vi "LabVIEW Task Manager.vi"() -> ()   [LabVIEW 2013]
doc: "Use this template to create an application that executes until you click the Stop button. Unlike the Single Loop Application VI that uses polling, this VI uses the Event Structure."
panel:
  in  "Data Tree":string[](tree)=["Get File Extension.vi"]
  in  "Timeout (ms)":i32=2000
  in  "vit":bool=TRUE
  in  "vi":bool
  in  "ctl":bool=TRUE
  in  "Open Front Panel":bool
  in  "Open Block Diagram":bool
  in  "Refresh":bool
  in  "Abort":bool
  # "Filter"
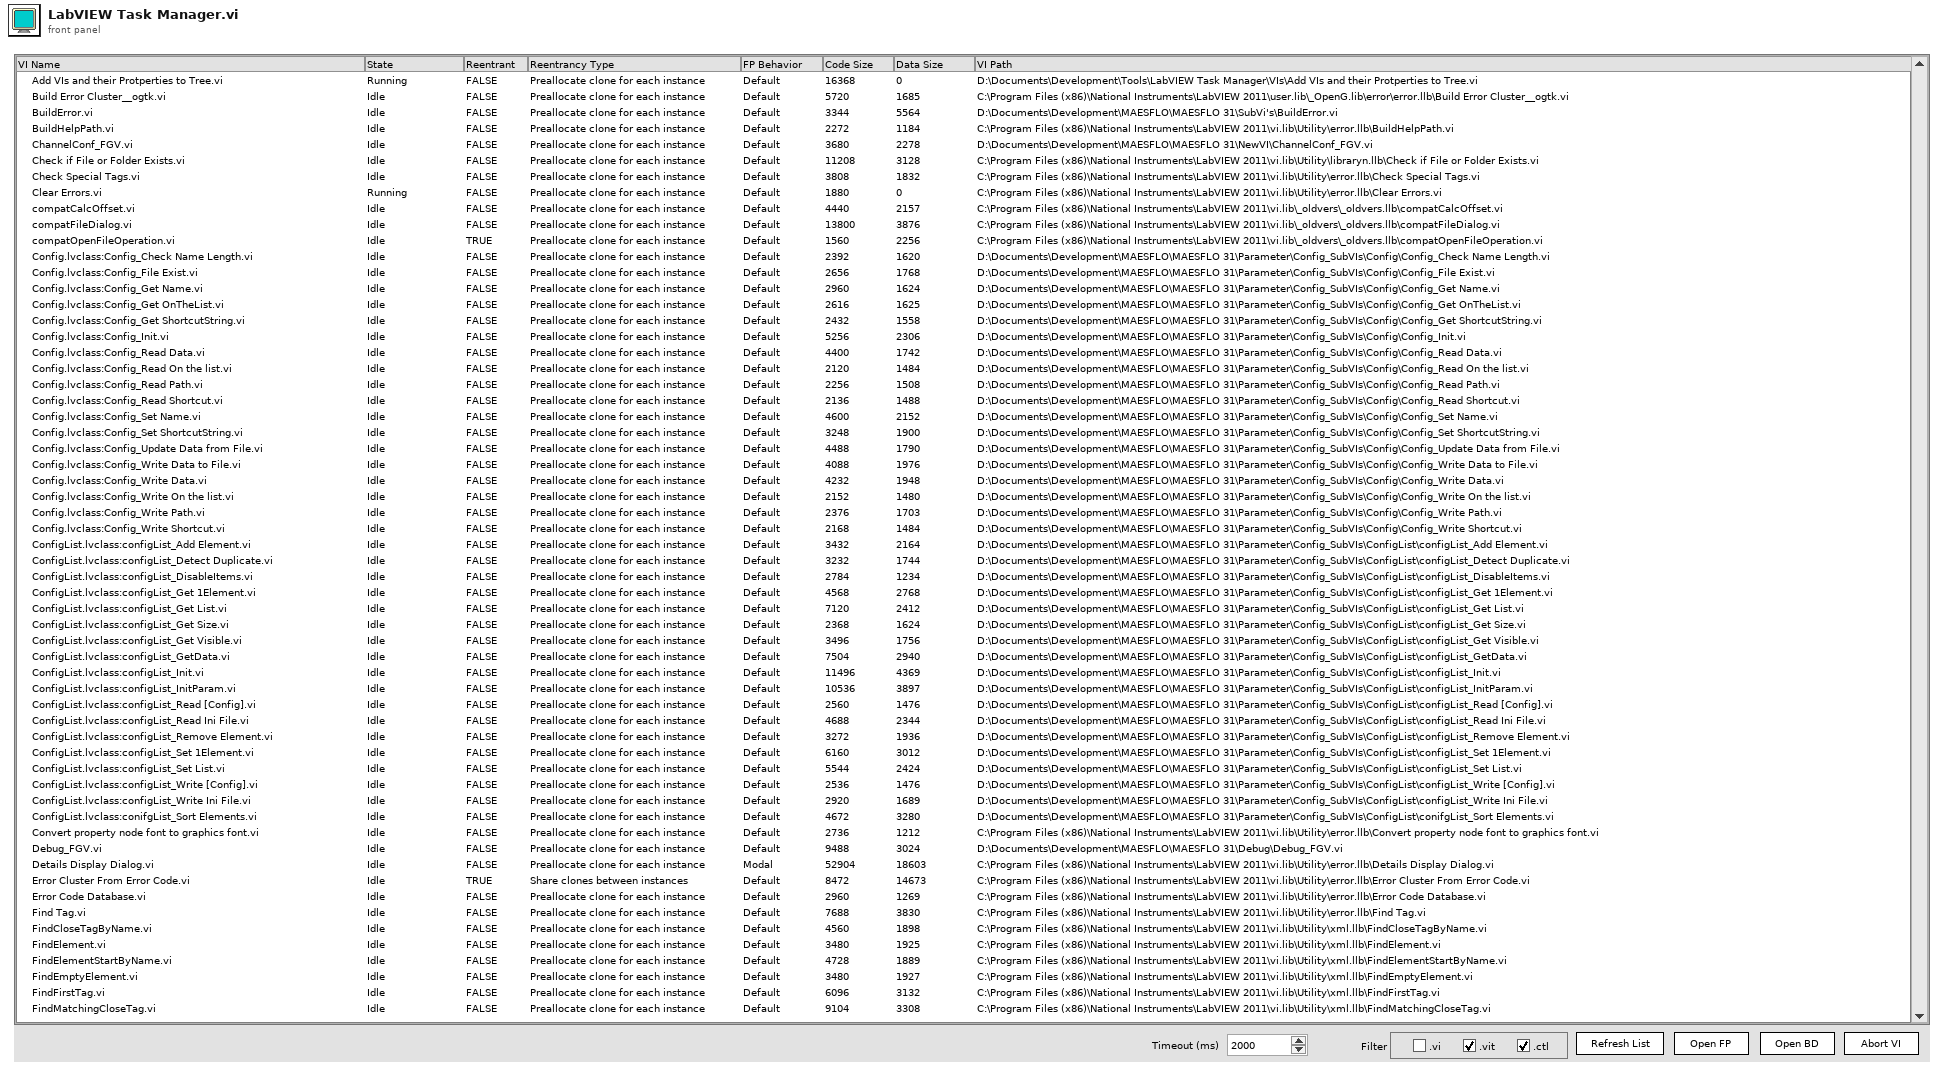
[diagram p1: front panel]
types:
  T1 = cluster{"Sort Column":i32, "Sorted AZ?":bool, "Data Tree Ref":refnum<vi>, "FP Ref":refnum<vi>, "Column Data Type":enum16{"String", "Numeric"}[]}
  T2 = enum32{"Bad", "Idle", "Run top level", "Running"}
  T3 = typedef "LVPoint32TypeDef.ctl" = cluster{"Horizontal":i32, "Vertical":i32}
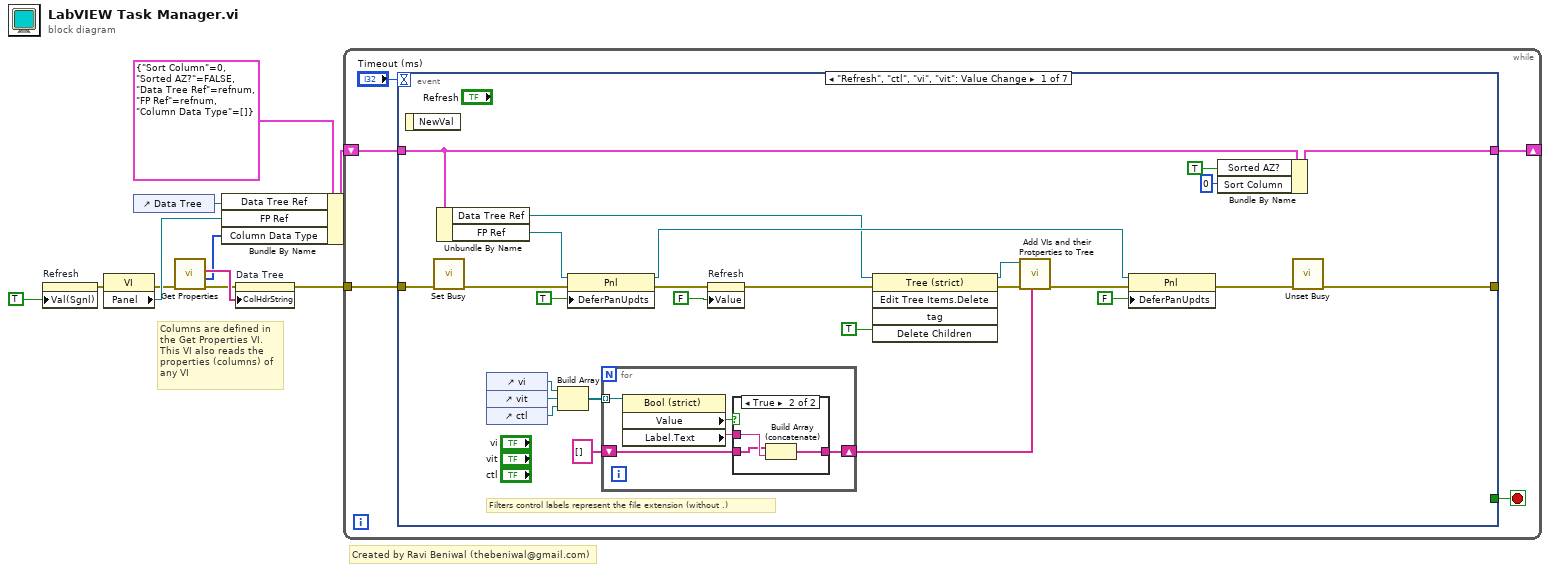
[diagram p0: block diagram]
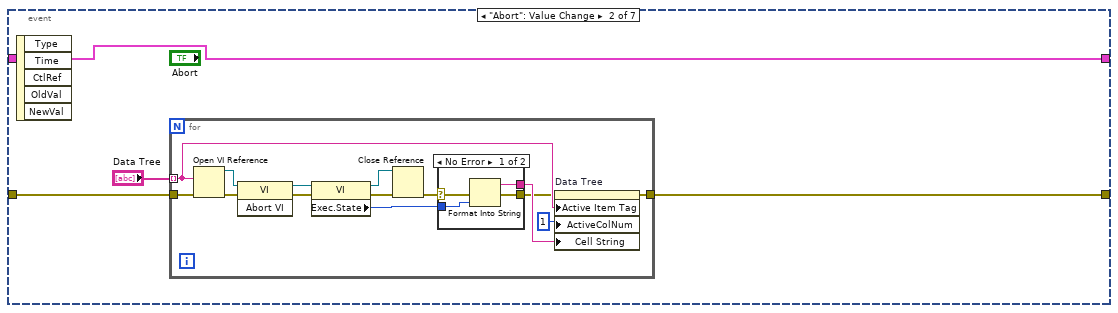
[diagram p3: hidden frame]
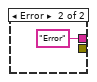
[diagram p4: hidden frame]
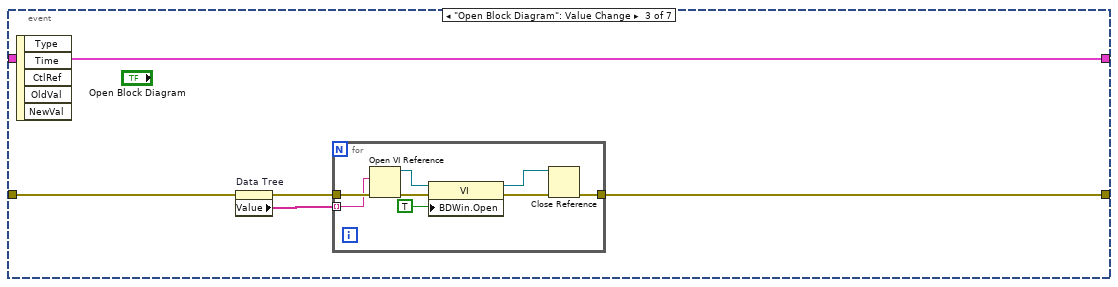
[diagram p5: hidden frame]
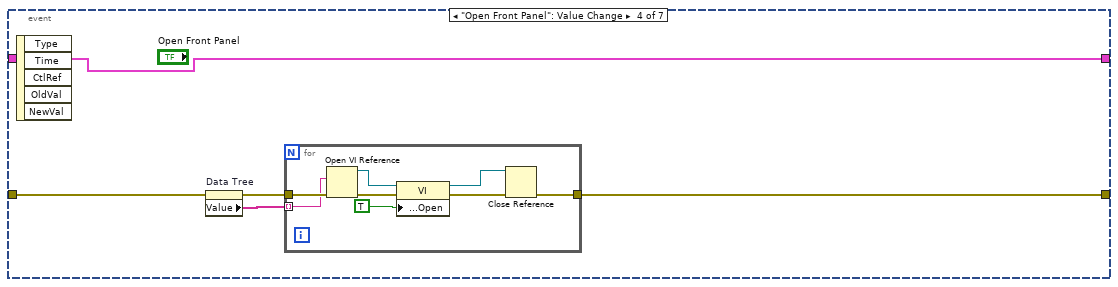
[diagram p6: hidden frame]
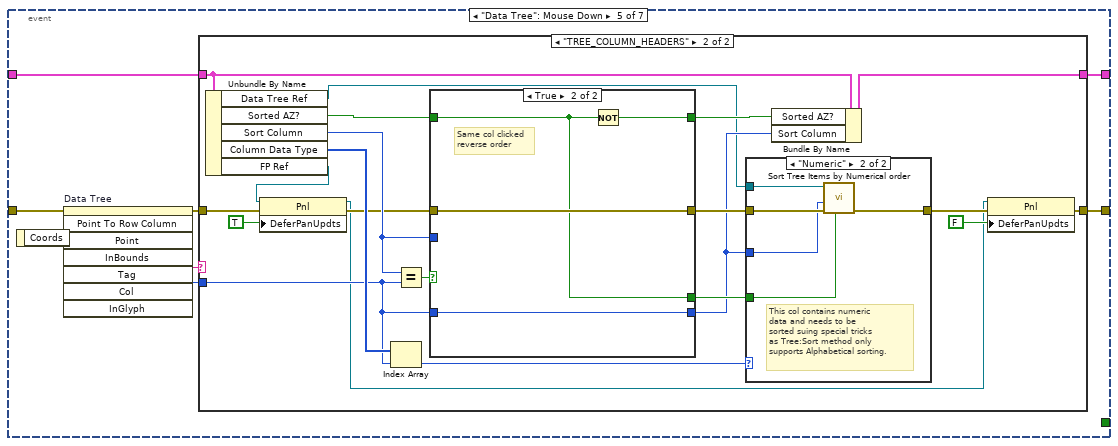
[diagram p7: hidden frame]
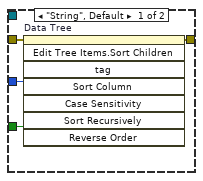
[diagram p9: hidden frame]
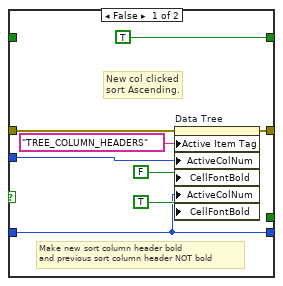
[diagram p10: hidden frame]
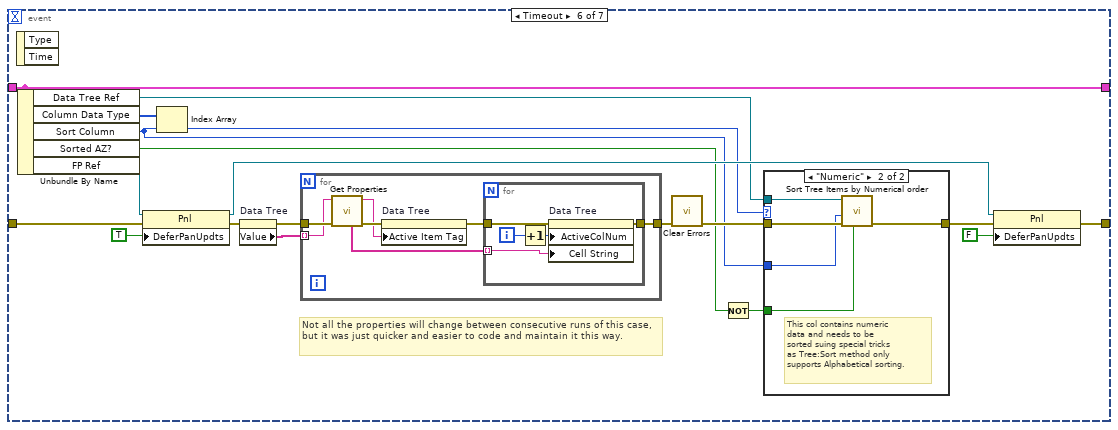
[diagram p11: hidden frame]
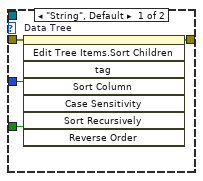
[diagram p12: hidden frame]
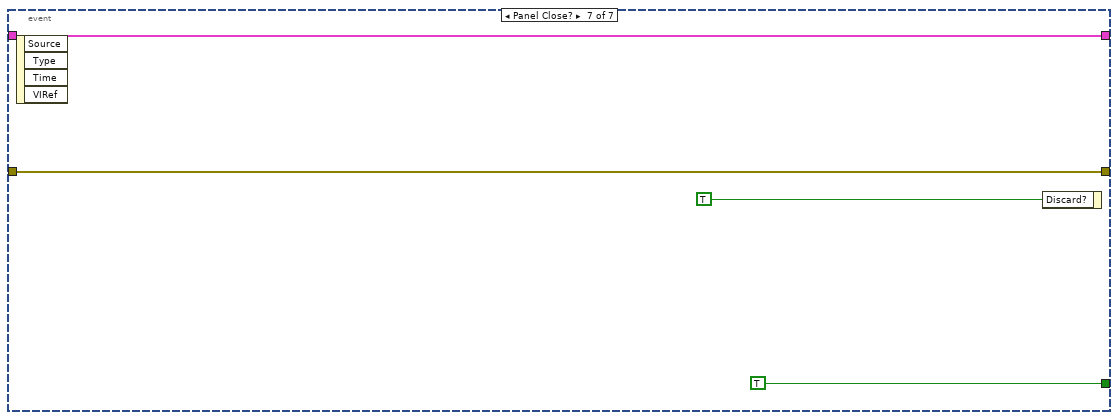
[diagram p13: hidden frame]
diagram:
  # "Columns are defined in the Get Properties VI. This VI also reads the properties (columns) of any VI"
  # "Created by Ravi Beniwal (thebeniwal@gmail.com)"
  n1 = property on="Refresh" class="Bool (strict)"("Val(Sgnl)"=TRUE ("Value (Signaling)")) -> (error out=w4:errorcluster)  [unwired: 2 in, 1 out]
  n2 = property class="VI"(error in=w4) -> (error out=w2:errorcluster, "Panel"=w5:refnum<vi>)  [unwired: 1 in, 1 out]
  n3 = control-ref of="Data Tree"() -> (w8:refnum<vi>)
  n4 = call "Get Properties.vi"("error in"=w2) -> ("error out"=w6:errorcluster, "Column Data Type"=w1:enum16{"String", "Numeric"}[], "Column Labels"=w7:string[])  [unwired: 6 in, 2 out]
  n5 = Bundle By Name(cluster=T1 {"Sort Column"=0, "Sorted AZ?"=FALSE, "Data Tree Ref"=refnum, "FP Ref"=refnum, "Column Data Type"=[]}, "Data Tree Ref"=w8, "FP Ref"=w5, "Column Data Type"=w1) -> (w9:T1)
  n6 = property on="Data Tree" class="Tree (strict)"(error in=w6, "ColHdrString"=w7) -> (error out=w3:errorcluster)  [unwired: 1 in, 1 out]
  n7 = while {
    tunnel: w3 -> [w15]
    shift-right: [w12] -> _
    shift-left: w9 -> [w13]
    stop <- w16 stop-if-true
    n8 = event shown="[0] \"Refresh\", \"ctl\", \"vi\", \"vit\": Value Change" {
      selector: _ -> [_ _ _ _ _ _ _]
      dyn-events: _ -> [_ _ _ _ _ _ _]
      timeout: "Timeout (ms)" -> [_ _ _ _ _ _ _]
      tunnel: [_ _ _ _ _ _ TRUE ("stop")] -> w16
      tunnel: [w33 w55 w78 w91 w103 w165 w195] -> _
      tunnel: w15 -> [w32 w54 w79 w92 w108 w167 w195]
      tunnel: w13 -> [w20 w52 w75 w88 w101 w153 w193]
      tunnel: [w23 w52 w75 w88 w102 w153 w193] -> w12
      event "Refresh", "ctl", "vi", "vit": Value Change {
        # "Filters control labels represent the file extension (without .)"
        n9 = event-data() -> ()  [unwired: 2 out]
        n10 = call <vilib>:"Set Busy.vi"("error in (no error)"=w32) -> ("error out"=w17:errorcluster)  [unwired: 9 in, 1 out]
        n11 = Unbundle By Name(w20) -> ("Data Tree Ref"=w19:refnum<vi>, "FP Ref"=w18:refnum<vi>)
        n12 = control-ref of="vi"() -> (w31:refnum<vi>)
        n13 = control-ref of="vit"() -> (w30:refnum<vi>)
        n14 = control-ref of="ctl"() -> (w29:refnum<vi>)
        n15 = Build Array(w31, w30, w29) -> (w28:refnum<vi>[])
        n16 = property class="Pnl"(reference=w18, error in=w17, "DeferPanUpdts"=TRUE ("Defer Panel Updates")) -> (reference out=w21:refnum<vi>, error out=w35:errorcluster)
        n17 = for {
          tunnel: w28 -> [w47] mode=indexing
          shift-right: [w43] -> w26
          shift-left: string[] [] -> [w44]
          n18 = property class="Bool (strict)"(reference=w47) -> ("Value"=w46:bool, "Label.Text"=w45:string)  [unwired: 1 in, 2 out]
          n19 = case shown="True" w46 {
            tunnel: w45 -> [_ w51]
            tunnel: w44 -> [w48 w50]
            tunnel: [w48 w49] -> w43
            frame False {
            }
            frame True {
              n20 = Build Array (concatenate)(w50, w51) -> (w49:string[])
            }
          }
        }
        n21 = property on="Refresh" class="Bool (strict)"(error in=w35, "Value"=FALSE ("Refresh")) -> (error out=w39:errorcluster)  [unwired: 1 in, 1 out]
        n22 = invoke class="Tree (strict)" method="Edit Tree Items.Delete"(reference=w19, error in=w39, "Delete Children"=TRUE ("Delete Children?")) -> (reference out=w40:refnum<vi>, error out=w41:errorcluster)  [unwired: 2 in, 3 out]
        n23 = call "Add VIs and their Protperties to Tree.vi"("File Extension Filters"=w26, "error in"=w41, "Data Tree"=w40) -> ("error out"=w22:errorcluster)  [unwired: 8 in]
        n24 = property class="Pnl"(reference=w21, error in=w22, "DeferPanUpdts"=FALSE ("Defer Panel Updates")) -> (error out=w34:errorcluster)  [unwired: 1 out]
        n25 = Bundle By Name(cluster=w20, "Sorted AZ?"=TRUE, "Sort Column"=0) -> (w23:T1)
        n26 = call <vilib>:"Unset Busy.vi"("error in (no error)"=w34) -> ("error out"=w33:errorcluster)  [unwired: 10 in]
      }
      event "Abort": Value Change {
        n27 = event-data() -> ()  [unwired: 6 out]
        n28 = for {
          tunnel: [w62] -> w55
          tunnel: w54 -> [w67]
          tunnel: "Data Tree" -> [w60] mode=indexing
          n29 = Open VI Reference(vi path=w60, error in (no error)=w67) -> (vi reference=w68:refnum<vi>, error out=w69:errorcluster)  [unwired: 4 out]
          n30 = invoke class="VI" method="Abort VI"(reference=w68, error in=w69) -> (reference out=w64:refnum<vi>, error out=w65:errorcluster)  [unwired: 1 in, 1 out]
          n31 = property class="VI"(reference=w64, error in=w65) -> (reference out=w63:refnum<vi>, error out=w58:errorcluster, "Exec.State"=w66:T2)
          n32 = Close Reference(reference=w63, error in (no error)=w58) -> (error out=w56:errorcluster)
          n33 = case shown="No Error" w56 {
            selector: w56 -> [w70 _]
            tunnel: w66 -> [w73 _]
            tunnel: [w72 "Error"] -> w61
            tunnel: [w71 _] -> w57
            frame No Error {
              n34 = Format Into String(error in=w70, w73) -> (resulting string=w72:string, error out=w71:errorcluster)  [unwired: 2 in]
            }
            frame Error {
            }
          }
          n35 = property on="Data Tree" class="Tree (strict)"(error in=w57, "Active Item Tag"=w60, "ActiveColNum"=1 ("Active Cell:Active Column Number"), "Cell String"=w61) -> (error out=w62:errorcluster)  [unwired: 1 in, 1 out]
        }
      }
      event "Open Block Diagram": Value Change {
        n36 = event-data() -> ()  [unwired: 6 out]
        n37 = property on="Data Tree" class="Tree (strict)"(error in=w79) -> (error out=w77:errorcluster, "Value"=w76:string[])  [unwired: 1 in, 1 out]
        n38 = for {
          tunnel: [w87] -> w78
          tunnel: w77 -> [w86]
          tunnel: w76 -> [w85] mode=indexing
          n39 = Open VI Reference(vi path=w85, error in (no error)=w86) -> (vi reference=w83:refnum<vi>, error out=w84:errorcluster)  [unwired: 4 out]
          n40 = property class="VI"(reference=w83, error in=w84, "BDWin.Open"=TRUE ("Block Diagram Window:Open")) -> (reference out=w82:refnum<vi>, error out=w81:errorcluster)
          n41 = Close Reference(reference=w82, error in (no error)=w81) -> (error out=w87:errorcluster)
        }
      }
      event "Open Front Panel": Value Change {
        n42 = event-data() -> ()  [unwired: 6 out]
        n43 = property on="Data Tree" class="Tree (strict)"(error in=w92) -> (error out=w90:errorcluster, "Value"=w89:string[])  [unwired: 1 in, 1 out]
        n44 = for {
          tunnel: [w100] -> w91
          tunnel: w90 -> [w99]
          tunnel: w89 -> [w98] mode=indexing
          n45 = Open VI Reference(vi path=w98, error in (no error)=w99) -> (vi reference=w96:refnum<vi>, error out=w97:errorcluster)  [unwired: 4 out]
          n46 = property class="VI"(reference=w96, error in=w97, "Front Panel.Open"=TRUE ("Block Diagram Window:Open")) -> (reference out=w95:refnum<vi>, error out=w94:errorcluster)
          n47 = Close Reference(reference=w95, error in (no error)=w94) -> (error out=w100:errorcluster)
        }
      }
      event "Data Tree": Mouse Down {
        n48 = event-data() -> ("Coords"=w107:T3)  [unwired: 1 out]
        n49 = invoke on="Data Tree" class="Tree (strict)" method="Point To Row Column"(error in=w108, "Point"=w107) -> (error out=w105:errorcluster, "Tag"=w106:string, "Col"=w104:i32)  [unwired: 6 in, 5 out]
        n50 = case shown="\"TREE_COLUMN_HEADERS\"" w106 {
          tunnel: w105 -> [w110 w117]
          tunnel: w104 -> [_ w121]
          tunnel: [w110 w112] -> w103
          tunnel: [w109 w130] -> w102
          tunnel: w101 -> [w109 w131]
          frame Default {
          }
          frame "TREE_COLUMN_HEADERS" {
            n51 = Unbundle By Name(w131) -> ("Data Tree Ref"=w119:refnum<vi>, "Sorted AZ?"=w128:bool, "Sort Column"=w123:i32, "Column Data Type"=w122:enum16{"String", "Numeric"}[], "FP Ref"=w115:refnum<vi>)
            n52 = property class="Pnl"(reference=w115, error in=w117, "DeferPanUpdts"=TRUE ("Defer Panel Updates")) -> (reference out=w111:refnum<vi>, error out=w116:errorcluster)
            n53 = Index Array(array=w122, index=w121) -> (element=w120:enum16{"String", "Numeric"})
            n54 = Equal?(x=w123, y=w121) -> (x = y?=w129:bool)
            n55 = case shown="True" w129 {
              tunnel: w128 -> [_ w150]
              tunnel: [TRUE ("Sorted AZ?") w149] -> w127
              tunnel: [_ w150] -> w126
              tunnel: w116 -> [w144 w152]
              tunnel: [w143 w152] -> w125
              tunnel: w121 -> [w142 w151]
              tunnel: [w142 w151] -> w124
              tunnel: w123 -> [w141 _]
              frame False {
                # "Make new sort column header bold\nand previous sort column header NOT bold"
                # "New col clicked\nsort Ascending."
                n56 = property on="Data Tree" class="Tree (strict)"(error in=w144, "Active Item Tag"="TREE_COLUMN_HEADERS" ("Active Item:Tag"), "ActiveColNum"=w141, "CellFontBold"=FALSE ("Active Cell:Cell Font:Bold"), "ActiveColNum"=w142, "CellFontBold"=TRUE ("Active Cell:Cell Font:Bold")) -> (error out=w143:errorcluster)  [unwired: 1 in, 1 out]
              }
              frame True {
                # "Same col clicked\nreverse order"
                n57 = Not(x=w150) -> (.not. x?=w149:bool)
              }
            }
            n58 = case shown="\"Numeric\"" w120 {
              tunnel: [w135 w139] -> w113
              tunnel: w126 -> [w134 w138]
              tunnel: w125 -> [w133 w140]
              tunnel: w124 -> [w132 w136]
              tunnel: w119 -> [_ w137]
              frame "String", Default {
                n59 = invoke on="Data Tree" class="Tree (strict)" method="Edit Tree Items.Sort Children"(error in=w133, "Sort Column"=w132, "Reverse Order"=w134) -> (error out=w135:errorcluster)  [unwired: 5 in, 7 out]
              }
              frame "Numeric" {
                # "This col contains numeric\ndata and needs to be\nsorted suing special tricks\nas Tree:Sort method only\nsupports Alphabetical sorting."
                n60 = call "Sort Tree Items by Numerical order.vi"("Reverse Order?"=w138, "error in"=w140, "Sort Column"=w136, "Data Tree"=w137) -> ("error out"=w139:errorcluster)  [unwired: 7 in]
              }
            }
            n61 = Bundle By Name(cluster=w131, "Sorted AZ?"=w127, "Sort Column"=w124) -> (w130:T1)
            n62 = property class="Pnl"(reference=w111, error in=w113, "DeferPanUpdts"=FALSE ("Defer Panel Updates")) -> (error out=w112:errorcluster)  [unwired: 1 out]
          }
        }
      }
      event Timeout {
        # "Not all the properties will change between consecutive runs of this case, but it was just quicker and easier to code and maintain it this way."
        n63 = event-data() -> ()  [unwired: 3 out]
        n64 = Unbundle By Name(w153) -> ("Data Tree Ref"=w159:refnum<vi>, "Column Data Type"=w158:enum16{"String", "Numeric"}[], "Sort Column"=w157:i32, "Sorted AZ?"=w156:bool, "FP Ref"=w162:refnum<vi>)
        n65 = property class="Pnl"(reference=w162, error in=w167, "DeferPanUpdts"=TRUE ("Defer Panel Updates")) -> (reference out=w164:refnum<vi>, error out=w166:errorcluster)
        n66 = Index Array(array=w158, index=w157) -> (element=w155:enum16{"String", "Numeric"})
        n67 = property on="Data Tree" class="Tree (strict)"(error in=w166) -> (error out=w171:errorcluster, "Value"=w170:string[])  [unwired: 1 in, 1 out]
        n68 = for {
          tunnel: w171 -> [w187]
          tunnel: w170 -> [w186] mode=indexing
          tunnel: [w181] -> w163
          n69 = call "Get Properties.vi"("error in"=w187, "VI Name"=w186) -> ("error out"=w185:errorcluster, "VI Name Out"=w184:string, "VI Properties"=w182:string[])  [unwired: 5 in, 2 out]
          n70 = property on="Data Tree" class="Tree (strict)"(error in=w185, "Active Item Tag"=w184) -> (error out=w183:errorcluster)  [unwired: 1 in, 1 out]
          n71 = for {
            tunnel: w183 -> [w192]
            tunnel: w182 -> [w189] mode=indexing
            tunnel: [w188] -> w181
            i -> [w191]
            n72 = Increment(x=w191) -> (x+1=w190:i32)
            n73 = property on="Data Tree" class="Tree (strict)"(error in=w192, "ActiveColNum"=w190, "Cell String"=w189) -> (error out=w188:errorcluster)  [unwired: 1 in, 1 out]
          }
        }
        n74 = call <vilib>:"Clear Errors.vi"("error in (no error)"=w163) -> ("error out"=w160:errorcluster)  [unwired: 6 in]
        n75 = Not(x=w156) -> (.not. x?=w154:bool)
        n76 = case shown="\"Numeric\"" w155 {
          tunnel: [w175 w179] -> w161
          tunnel: w154 -> [w174 w178]
          tunnel: w160 -> [w173 w180]
          tunnel: w157 -> [w172 w176]
          tunnel: w159 -> [_ w177]
          frame "String", Default {
            n77 = invoke on="Data Tree" class="Tree (strict)" method="Edit Tree Items.Sort Children"(error in=w173, "Sort Column"=w172, "Reverse Order"=w174) -> (error out=w175:errorcluster)  [unwired: 5 in, 7 out]
          }
          frame "Numeric" {
            # "This col contains numeric\ndata and needs to be\nsorted suing special tricks\nas Tree:Sort method only\nsupports Alphabetical sorting."
            n78 = call "Sort Tree Items by Numerical order.vi"("Reverse Order?"=w178, "error in"=w180, "Sort Column"=w176, "Data Tree"=w177) -> ("error out"=w179:errorcluster)  [unwired: 7 in]
          }
        }
        n79 = property class="Pnl"(reference=w164, error in=w161, "DeferPanUpdts"=FALSE ("Defer Panel Updates")) -> (error out=w165:errorcluster)  [unwired: 1 out]
      }
      event Panel Close? {
        n80 = event-data() -> ()  [unwired: 5 out]
        n81 = event-data("Discard?"=TRUE) -> ()  [unwired: 1 in, 1 out]
      }
    }
  }
